vi "MODAQ Send Mail (subvi).vi"(1 "Message":string, 2 "Subject":string, 3 "To":string[](array[string])) -> (0 "error out":errorcluster)   [LabVIEW 2019]
uses:
  Globals and Definitions/Initialization Globals.vi
  <vilib>/smtpClient/Set Message Text.vi
  <vilib>/smtpClient/LabVIEWSMTPClient.lvlib
panel:
  out "invalid recipients":string[](array[string])
  in  "Port":string="587"
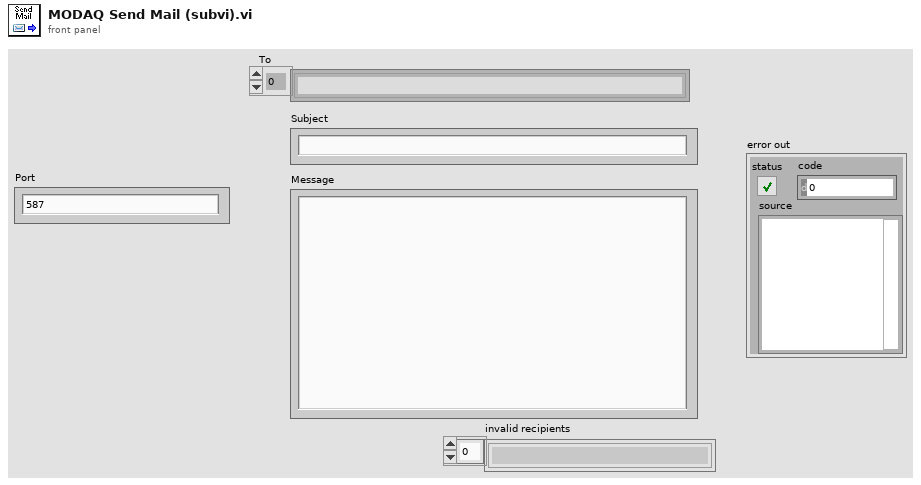
[diagram p1: front panel]
types:
  T1 = typedef "LabVIEWSMTPClient.lvlib/SmtpClientHandle.ctl" = refnum<k1>
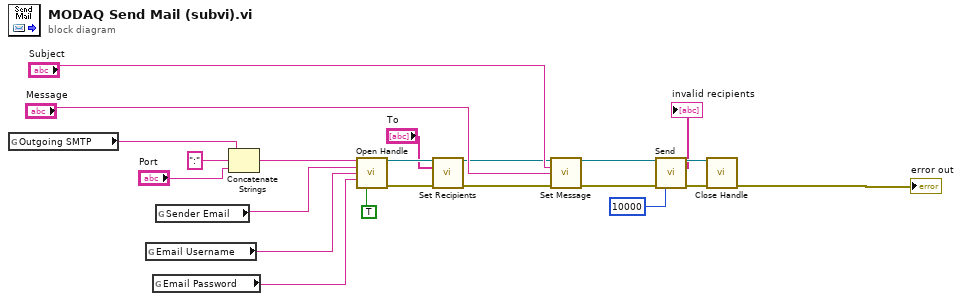
[diagram p0: block diagram]
diagram:
  n1 = global read "Initialization Globals.vi" "Outgoing SMTP"() -> (w4:string)
  n2 = global read "Initialization Globals.vi" "Email Username"() -> (w3:string)
  n3 = global read "Initialization Globals.vi" "Email Password"() -> (w2:string)
  n4 = global read "Initialization Globals.vi" "Sender Email"() -> (w5:string)
  n5 = Concatenate Strings(w4, ":" ("string"), "Port") -> (w8:string)
  n6 = call <vilib>:"Open Handle.vi"("server address"=w8, "from"=w5, "username"=w3, "password"=w2, "use TLS (false)"=TRUE ("Enable TLS")) -> ("handle out"=w16:T1, "error out"=w17:errorcluster)  [unwired: 9 in]
  n7 = call <vilib>:"Set Recipients.vi"("handle in"=w16, "to"="To", "error in (no error)"=w17) -> ("handle out"=w13:T1, "error out"=w14:errorcluster)  [unwired: 11 in]
  n8 = call-poly <vilib>:"Set Message.vi"("handle in"=w13, "subject"="Subject", "plain text message"="Message", "error in (no error)"=w14) -> ("handle out"=w11:T1, "error out"=w12:errorcluster)  [unwired: 10 in]
  n9 = call <vilib>:"Send.vi"("handle in"=w11, "error in (no error)"=w12, "timeout in ms (10000)"=10000 ("timeout in ms")) -> ("handle out"=w18:T1, "invalid recipients"=→"invalid recipients":string[], "error out"=w19:errorcluster)  [unwired: 10 in]
  n10 = call <vilib>:"Close Handle.vi"("handle in"=w18, "error in (no error)"=w19) -> ("error out"=→"error out":errorcluster)  [unwired: 12 in, 1 out]
